vi "PLL data source -- SRS860.vi"(6 "set-get delay (msec)":i64, 7 "data source action":T2=enum."get", 9 "z  in (V)":cdb, 10 "Freq in (Hz)":dbl=40000.0 format="%#_13g", 11 "PLL data source":T1=enum."SRS865A") -> (1 "z out (V)":cdb=0.00010527635459-2.9308681405e-05i, 2 "Freq out (Hz)":dbl=55115.2, 3 "PLL data source OUT":T1=enum."SRS865A")   [LabVIEW 2018]
uses:
  PLL data source.ctl
  data source action.ctl
  publisher action.ctl
  <instrlib>/Stanford Research SR865/Public/Utility/Error Query.vi
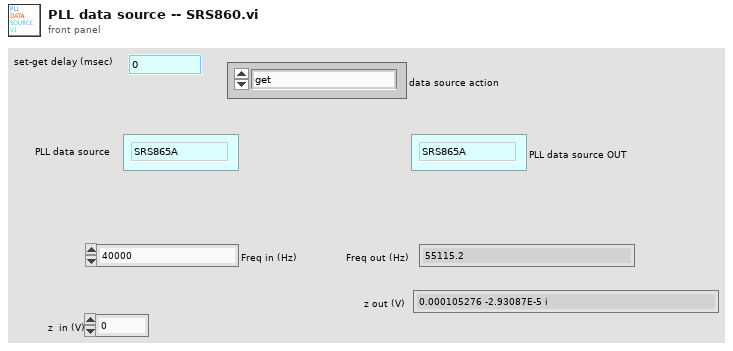
[diagram p1: front panel]
types:
  T1 = typedef "PLL data source.ctl" = enum16{"meta", "MFLI", "SRS865A"}
  T2 = typedef "data source action.ctl" = enum16{"set", "get", "init", "set-and-get"}
  T3 = typedef "publisher action.ctl" = enum16{"set", "get", "init", "check"}
  T4 = typedef "Zurich Instruments LabOne.lvlib/ziTypeHandle.ctl" = cluster{"handleValid":bool, "Conn":u64, "Path Prefix":string, "Handle":u64, "Connected":bool, "Clockbase(s)":dbl}
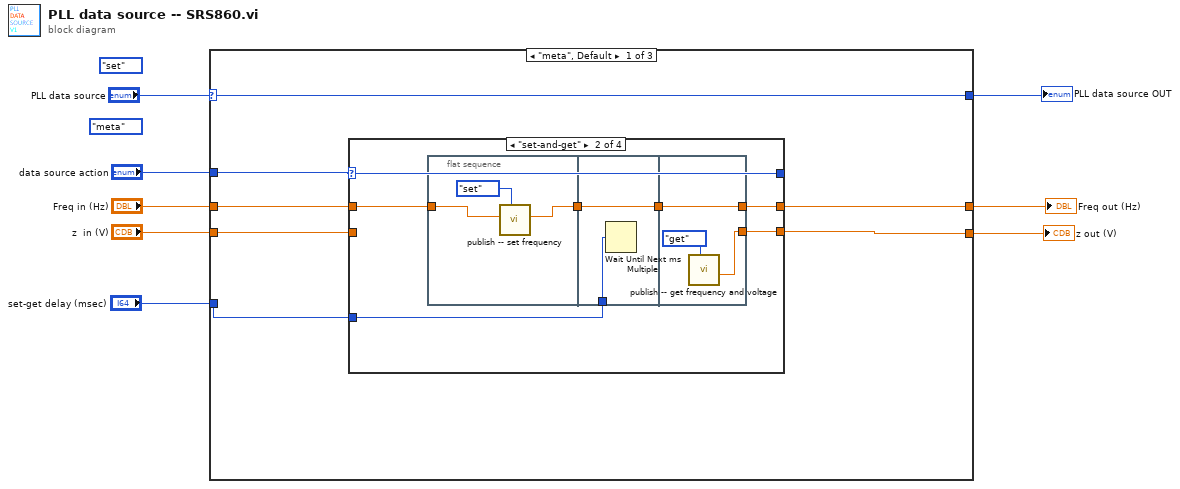
[diagram p0: block diagram]
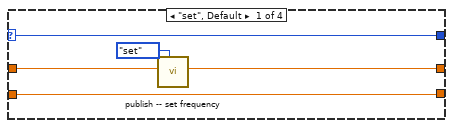
[diagram p2: hidden frame]
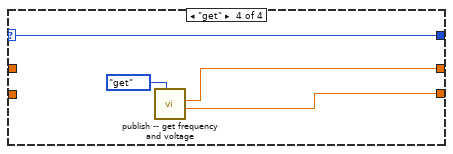
[diagram p4: hidden frame]
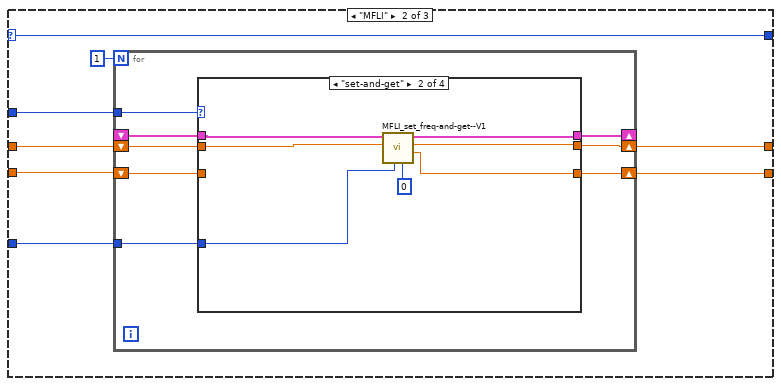
[diagram p5: hidden frame]
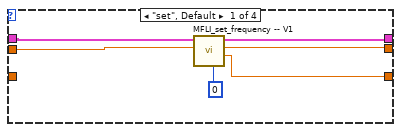
[diagram p6: hidden frame]
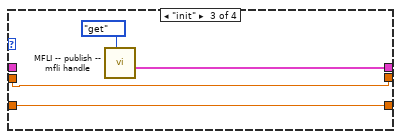
[diagram p7: hidden frame]
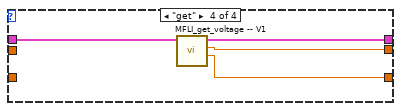
[diagram p8: hidden frame]
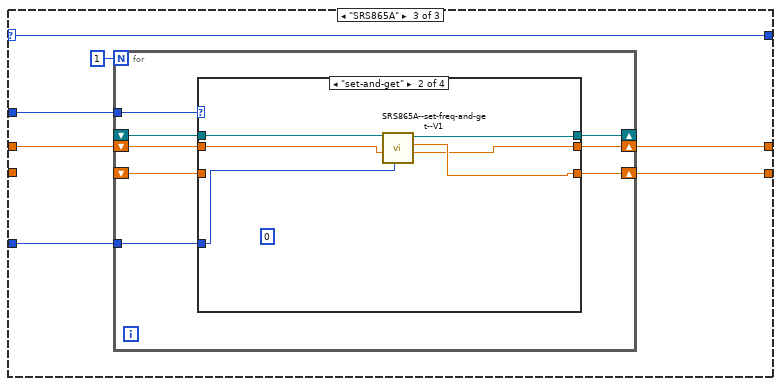
[diagram p9: hidden frame]
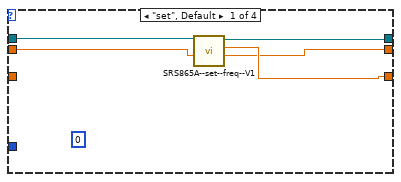
[diagram p10: hidden frame]
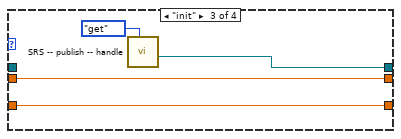
[diagram p11: hidden frame]
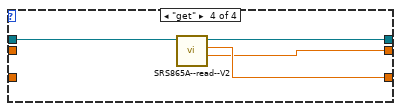
[diagram p12: hidden frame]
diagram:
  (unwired) data_source_action."set" ("data source action")
  (unwired) PLL_data_source."meta" ("PLL data source")
  n1 = case shown="\"meta\", Default" "PLL data source" {
    selector: "PLL data source" -> [w12 w47 w83]
    tunnel: "data source action" -> [w13 w46 w82]
    tunnel: [w14 w50 w86] -> w6
    tunnel: "Freq in (Hz)" -> [w15 w49 w85]
    tunnel: [w12 w47 w83] -> w4
    tunnel: "set-get delay (msec)" -> [w11 w45 w81]
    tunnel: "z  in (V)" -> [w9 w44 _]
    tunnel: [w10 w43 w80] -> w1
    frame "meta", Default {
      n2 = case shown="\"set-and-get\"" w13 {
        selector: w13 -> [w17 w25 w37 w40]
        tunnel: [w18 w26 w38 w41] -> w14
        tunnel: w15 -> [w19 w27 w38 _]
        tunnel: [w17 w25 w37 w40] -> _
        tunnel: w11 -> [_ w22 _ _]
        tunnel: [w16 w21 w36 w39] -> w10
        tunnel: w9 -> [w16 _ w36 _]
        frame "set", Default {
          n3 = call "publish -- set frequency.vi"("publisher action"=publisher_action."set", "freq IN (Hz)"=w19) -> ("freq out (Hz)"=w18:dbl)  [unwired: 9 in]
        }
        frame "set-and-get" {
          n4 = flat-sequence {
            tunnel: w27 -> [w29]
            tunnel: [w28] -> w24
            tunnel: w24 -> [w32]
            tunnel: [w32] -> w23
            tunnel: w22 -> [w31]
            tunnel: [w35] -> w26
            tunnel: w23 -> [w35]
            tunnel: [w33] -> w21
            frame #0 {
              n5 = call "publish -- set frequency.vi"("publisher action"=publisher_action."set", "freq IN (Hz)"=w29) -> ("freq out (Hz)"=w28:dbl)  [unwired: 9 in]
            }
            frame #1 {
              n6 = Wait Until Next ms Multiple(millisecond multiple=w31) -> ()  [unwired: 1 out]
            }
            frame #2 {
              n7 = call "publish -- get frequency and voltage.vi"("publisher action"=publisher_action."get") -> ("Voltage out (V)"=w33:cdb)  [unwired: 8 in, 2 out]
            }
          }
        }
        frame "init" {
        }
        frame "get" {
          n8 = call "publish -- get frequency and voltage.vi"("publisher action"=publisher_action."get") -> ("Voltage out (V)"=w39:cdb, "freq out (Hz)"=w41:dbl)  [unwired: 8 in, 1 out]
        }
      }
    }
    frame "MFLI" {
      n9 = for {
        N: 1 -> [_]
        shift-right: [w58] -> _
        shift-left: _ -> [w57]
        shift-right: [w56] -> w50
        shift-left: w49 -> [w54]
        shift-right: [w55] -> w43
        shift-left: w44 -> [w53]
        tunnel: w46 -> [w52]
        tunnel: w45 -> [w51]
        n10 = case shown="\"set-and-get\"" w52 {
          tunnel: [w64 w71 w74 w79] -> w58
          tunnel: w57 -> [w63 w70 _ w78]
          tunnel: [w60 w67 w72 w77] -> w56
          tunnel: [w59 w66 w73 w76] -> w55
          tunnel: w54 -> [w61 w68 w72 _]
          tunnel: w53 -> [_ _ w73 _]
          tunnel: w51 -> [_ w65 _ _]
          frame "set", Default {
            n11 = call "MFLI_set_frequency -- V1.vi"("Oscillator (0)"=u16 0, "Freq in (Hz)"=w61, "Handle In"=w63) -> ("z out (V)"=w59:cdb, "Freq out (Hz)"=w60:dbl, "Handle Out"=w64:T4)  [unwired: 5 in, 1 out]
          }
          frame "set-and-get" {
            n12 = call "MFLI_set_freq-and-get--V1.vi"("Oscillator (0)"=u16 0, "delay-circle(msec)"=w65, "Freq in (Hz)"=w68, "Handle In"=w70) -> ("z out (V)"=w66:cdb, "Freq out (Hz)"=w67:dbl, "Handle Out"=w71:T4)  [unwired: 4 in, 1 out]
          }
          frame "init" {
            n13 = call "MFLI -- publish -- mfli handle.vi"("publisher action"=publisher_action."get") -> ("Handle Out"=w74:T4)  [unwired: 10 in]
          }
          frame "get" {
            n14 = call "MFLI_get_voltage -- V1.vi"("Handle In"=w78) -> ("z out (V)"=w76:cdb, "Freq out (Hz)"=w77:dbl, "Handle Out"=w79:T4)  [unwired: 7 in, 1 out]
          }
        }
      }
    }
    frame "SRS865A" {
      n15 = for {
        N: 1 -> [_]
        shift-right: [w94] -> _
        shift-left: _ -> [w93]
        shift-right: [w89] -> w86
        shift-left: w85 -> [w88]
        shift-right: [w92] -> w80
        shift-left: _ -> [w91]
        tunnel: w82 -> [w90]
        tunnel: w81 -> [w87]
        n16 = case shown="\"set-and-get\"" w90 {
          tunnel: [w98 w104 w108 w111] -> w94
          tunnel: w93 -> [w99 w105 _ w112]
          tunnel: [w97 w103 w107 w113] -> w92
          tunnel: w91 -> [_ _ w107 _]
          tunnel: [w96 w102 w106 w110] -> w89
          tunnel: w88 -> [w95 w101 w106 _]
          tunnel: w87 -> [_ w100 _ _]
          frame "set", Default {
            (unwired) u16 0 ("Oscillator (0)")
            n17 = call "SRS865A--set--freq--V1.vi"("freq in"=w95, "VISA resource name"=w99) -> ("freq out"=w96:dbl, "zi out (V)"=w97:cdb, "VISA resource name out"=w98:refnum<visa-resource-name>)  [unwired: 6 in, 1 out]
          }
          frame "set-and-get" {
            (unwired) u16 0 ("Oscillator (0)")
            n18 = call "SRS865A--set-freq-and-get--V1.vi"("delay-circle(msec)"=w100, "freq in"=w101, "VISA resource name"=w105) -> ("freq out"=w102:dbl, "zi out (V)"=w103:cdb, "VISA resource name out"=w104:refnum<visa-resource-name>)  [unwired: 5 in, 1 out]
          }
          frame "init" {
            n19 = call "SRS -- publish -- handle.vi"("publisher action"=publisher_action."get") -> ("SRS865 visa OUT"=w108:refnum<visa-resource-name>)  [unwired: 10 in]
          }
          frame "get" {
            n20 = call "SRS865A--read--V2.vi"("VISA resource name"=w112) -> ("freq out"=w110:dbl, "zi out (V)"=w113:cdb, "VISA resource name out"=w111:refnum<visa-resource-name>)  [unwired: 7 in, 1 out]
          }
        }
      }
    }
  }
  "Freq out (Hz)" <- w6
  "z out (V)" <- w1
  "PLL data source OUT" <- w4
